vi "Simulation VI.vi"() -> ()   [LabVIEW 2014]
uses:
  <vilib>/rvi/DesktopExecutionNode/Execution/niFpgaDEN_Execute.vi
  <vilib>/rvi/DesktopExecutionNode/DesktopExecutionNode.xnode
panel:
  out "Digital Waveform Graph":digitaldata(graph)
  in  "Connector0/DIO1":bool
  in  "stop":bool
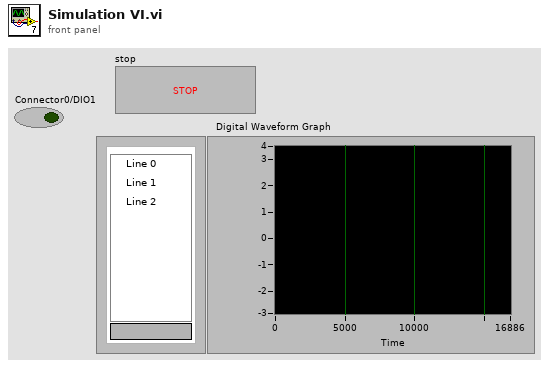
[diagram p1: front panel]
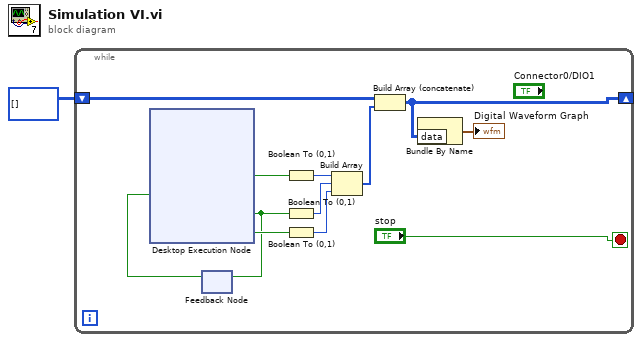
[diagram p0: block diagram]
diagram:
  n1 = while {
    shift-right: [w8] -> _
    shift-left: i16[][] [] -> [w7]
    stop <- "stop" stop-if-true
    n2 = feedback #1() -> (w3:bool)  [unwired: 1 in]
    n3 = xnode "Desktop Execution Node"("Connector0/DIO1"=w3) -> ("Connector0/DIO0"=w5:bool, "Connector0/DIO2"=w2:bool, "Connector0/DIO3"=w4:bool)  [unwired: 1 in, 1 out]
    n4 = feedback-in #1(w2) -> ()
    n5 = Boolean To (0,1)(Boolean=w5) -> (0, 1=w12:i16)
    n6 = Boolean To (0,1)(Boolean=w2) -> (0, 1=w11:i16)
    n7 = Boolean To (0,1)(Boolean=w4) -> (0, 1=w10:i16)
    n8 = Build Array(w12, w11, w10) -> (w9:i16[])
    n9 = Build Array (concatenate)(w7, w9) -> (w8:i16[][])
    n10 = Bundle By Name("data"=w8) -> (→"Digital Waveform Graph":digitaldata)  [unwired: 1 in]
  }
